vi "Handle Command.vi"(8 "error in (no error)":errorcluster, 9 "Value":bool, 11 "Valve in":refnum<class "MultiControl.lvclass">) -> (0 "error out":errorcluster, 3 "Valve out":refnum<class "MultiControl.lvclass">)   [LabVIEW 2020, in "VolatusControl.lvlib" / "MultiControl.lvclass"]
uses:
  MultiControl.lvclass
  MultiControl.lvclass/MultiControl.ctl
  messages/CmdDigitalMultiple/Data.ctl
  messages/CmdDigital/Data.ctl
  Volatus/MessageQ/MessageQ.lvclass/MessageQ.ctl
  Volatus/MessageQ/MessageQ.lvclass
  messages/CmdDigital/CmdDigital.lvlib
  messages/CmdDigitalMultiple/CmdDigitalMultiple.lvlib
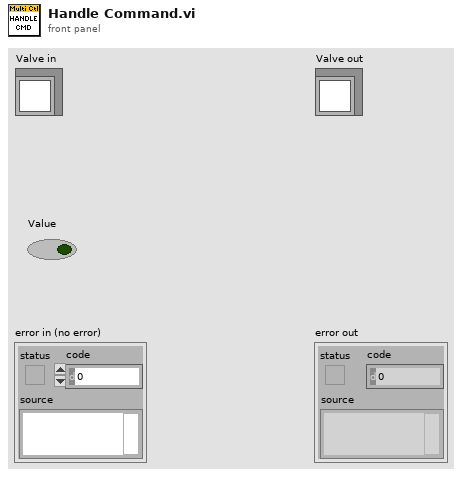
[diagram p1: front panel]
types:
  T1 = typedef "CmdDigitalMultiple.lvlib/Data.ctl" = cluster{"values":T2[]}
  T2 = typedef "CmdDigital.lvlib/Data.ctl" = cluster{"channel":string, "value":bool}
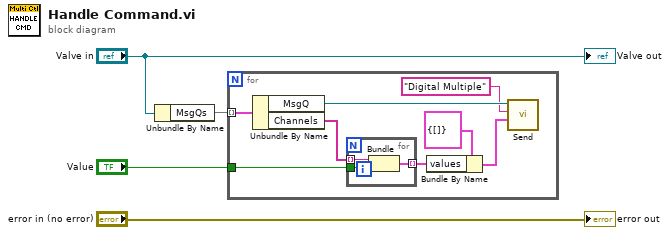
[diagram p0: block diagram]
diagram:
  n1 = Unbundle By Name("Valve in") -> ("MsgQs"=w1:map{refnum<class "MessageQ.lvclass">, string[]})
  n2 = for {
    tunnel: "Value" -> [w7]
    tunnel: w1 -> [w12] mode=indexing
    n3 = Unbundle By Name(w12) -> ("MsgQ"=w11:refnum<class "MessageQ.lvclass">, "Channels"=w9:string[])
    n4 = for {
      tunnel: w9 -> [w15] mode=indexing
      tunnel: [w14] -> w8 mode=indexing
      tunnel: w7 -> [w13]
      n5 = Bundle("String"=w15, "Value"=w13) -> (w14:cluster{"String":string, "Value":bool})  [unwired: 1 in]
    }
    n6 = Bundle By Name(cluster=T1 {"values"=[]} ("input cluster"), "values"=w8) -> (w6:T1)
    n7 = call "Send.vi"("Data"=w6, "ID"="Digital Multiple", "MessageQ in"=w11) -> ()  [unwired: 7 in, 2 out]
  }
  "error out" <- "error in (no error)"
  "Valve out" <- "Valve in"
